vi "Rate to Sampls&Time.vi"(8 "error in (no error)":errorcluster, 10 "JSON Cluster":T1, 11 "Select Update Rate":enum16{"HIGH", "MEDIUM", "LOW"}(ring)) -> (0 "error out":errorcluster, 2 "TimeElapsed":i32, 3 "SampleElapsed":i32)   [LabVIEW 2019, in "Zen Analytics.lvlib" / "Zen Analytics.lvclass"]
uses:
  Zen Analytics.lvclass
  Dependency/JSON Cluster(Int).ctl
types:
  T1 = typedef "Zen Analytics.lvlib/Zen Analytics.lvclass/JSON Cluster(Int).ctl" = cluster{"Rows In 2D Array":i32, "Columns In 2D Array":i32, "Samples To Display":i32, "Update Rate (Time)":i32, "Update Rate (Samples)":i32, "CurrentPartNumber":string, "AnalyticsDataFormat":cluster{"AnalyticsParameters":cluster{"UpdateRateCategories":cluster{"LOW":cluster{"SampleElapsed":dbl, "TimeElapsed":dbl}, "MEDIUM":cluster{"SampleElapsed":dbl, "TimeElapsed":dbl}, "HIGH":cluster{"SampleElapsed":dbl, "TimeElapsed":dbl}}, "AnalyticsForPartsList":cluster{"Name":string, "InitializationValues":cluster{"RowsIn2DArray":dbl, "ColumnsIn2DArray":dbl, "SamplesToDisplay":dbl, "UpdateRate":string}, "PlotParameters":cluster{"Trend":cluster{"TrendPlotID":dbl, "PlotProperties":cluster{"FontName":string, "FontSize":dbl, "FontColor":string, "IsBold":bool, "IsItalic":bool, "PlotColor":string}}[], "Histogram":cluster{"HistogramPlotID":dbl, "PlotProperties":cluster{"FontName":string, "FontSize":dbl, "FontColor":string, "IsBold":bool, "IsItalic":bool, "PlotColor":string}}[], "BarPlot":cluster{"BarPlotID":dbl, "BarValuesID":dbl, "PlotProperties":cluster{"FontName":string, "FontSize":dbl, "IsBold":bool, "IsItalic":bool, "FontColor":string}, "Sectors":string[]}[], "PieChart":cluster{"PieChartID":dbl, "PieChartValueID":dbl, "PlotProperties":cluster{"FontName":string, "FontSize":dbl, "IsBold":bool, "IsItalic":bool, "FontColor":string}, "Sectors":string[]}[]}}[]}}, "MeasurementData":cluster{"Measurement ID":i32, "Measurement Name":string, "Nominal Values":dbl, "LSL":dbl, "USL":dbl, "LCL":dbl, "UCL":dbl}[], "PlotParameters":cluster{"Trend":cluster{"TrendPlotID":dbl, "PlotProperties":cluster{"FontName":string, "FontSize":dbl, "FontColor":string, "IsBold":bool, "IsItalic":bool, "PlotColor":string}}[], "Histogram":cluster{"HistogramPlotID":dbl, "PlotProperties":cluster{"FontName":string, "FontSize":dbl, "FontColor":string, "IsBold":bool, "IsItalic":bool, "PlotColor":string}}[], "BarPlot":cluster{"BarPlotID":dbl, "BarValuesID":dbl, "PlotProperties":cluster{"FontName":string, "FontSize":dbl, "IsBold":bool, "IsItalic":bool, "FontColor":string}, "Sectors":string[]}[], "PieChart":cluster{"PieChartID":dbl, "PieChartValueID":dbl, "PlotProperties":cluster{"FontName":string, "FontSize":dbl, "IsBold":bool, "IsItalic":bool, "FontColor":string}, "Sectors":string[]}[]}}
  T2 = cluster{"LOW":cluster{"SampleElapsed":dbl, "TimeElapsed":dbl}, "MEDIUM":cluster{"SampleElapsed":dbl, "TimeElapsed":dbl}, "HIGH":cluster{"SampleElapsed":dbl, "TimeElapsed":dbl}}
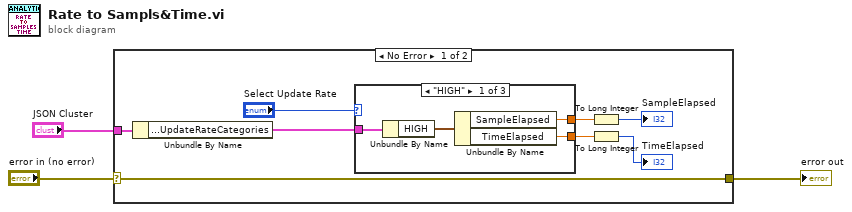
[diagram p0: block diagram]
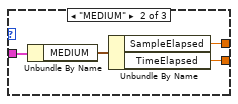
[diagram p2: hidden frame]
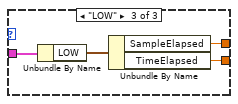
[diagram p3: hidden frame]
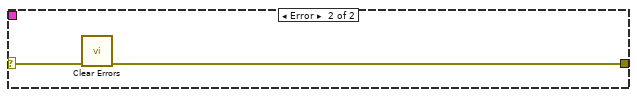
[diagram p4: hidden frame]
diagram:
  n1 = case shown="No Error" "error in (no error)" {
    selector: "error in (no error)" -> [w8 w25]
    tunnel: [w8 w24] -> w1
    tunnel: "JSON Cluster" -> [w7 _]
    frame No Error {
      n2 = Unbundle By Name(w7) -> ("AnalyticsDataFormat.AnalyticsParameters.UpdateRateCategories"=w6:T2)
      n3 = case shown="\"HIGH\"" "Select Update Rate" {
        tunnel: w6 -> [w15 w19 w23]
        tunnel: [w13 w17 w21] -> w10
        tunnel: [w12 w16 w20] -> w9
        frame "HIGH" {
          n4 = Unbundle By Name(w15) -> ("HIGH"=w14:cluster{"SampleElapsed":dbl, "TimeElapsed":dbl})
          n5 = Unbundle By Name(w14) -> ("SampleElapsed"=w13:dbl, "TimeElapsed"=w12:dbl)
        }
        frame "MEDIUM" {
          n6 = Unbundle By Name(w19) -> ("MEDIUM"=w18:cluster{"SampleElapsed":dbl, "TimeElapsed":dbl})
          n7 = Unbundle By Name(w18) -> ("SampleElapsed"=w17:dbl, "TimeElapsed"=w16:dbl)
        }
        frame "LOW" {
          n8 = Unbundle By Name(w23) -> ("LOW"=w22:cluster{"SampleElapsed":dbl, "TimeElapsed":dbl})
          n9 = Unbundle By Name(w22) -> ("SampleElapsed"=w21:dbl, "TimeElapsed"=w20:dbl)
        }
      }
      n10 = To Long Integer(number=w10) -> (32bit integer=→"SampleElapsed":i32)
      n11 = To Long Integer(number=w9) -> (32bit integer=→"TimeElapsed":i32)
    }
    frame Error {
      n12 = call <vilib>:"Clear Errors.vi"("error in (no error)"=w25) -> ("error out"=w24:errorcluster)  [unwired: 5 in, 1 out]
    }
  }
  "error out" <- w1
